vi "ShootAuto.vi"(8 "error in (no error)":errorcluster, 11 "Shooter":dbl) -> (0 "error out":errorcluster)   [LabVIEW 2012]
uses:
  Robot Global Data.vi
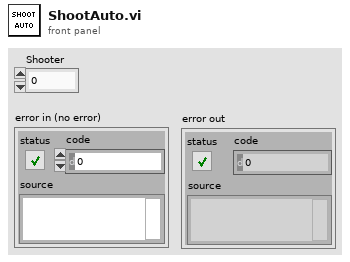
[diagram p1: front panel]
types:
  T1 = cluster{"Shoot":bool, "Enable_Targeting":bool, "Shooter":dbl, "LeadScrew":dbl, "Feed":bool, "Pickup":bool, "LiftHooks":bool, "Vision On":bool, "Vision Off":bool, "DownHooks":bool}
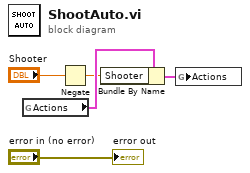
[diagram p0: block diagram]
diagram:
  n1 = global read "Robot Global Data.vi" "Actions"() -> (w4:T1)
  n2 = Negate(x="Shooter") -> (-x=w1:dbl)
  n3 = Bundle By Name(cluster=w4, "Shooter"=w1) -> (w5:T1)
  n4 = global write "Robot Global Data.vi" "Actions"(w5) -> ()
  "error out" <- "error in (no error)"
